vi "Get Bundler Input Terminal By Name.vi"(8 "error in (no error)":errorcluster, 10 "Terminal name":string, 11 "Bundler in":refnum<vi>) -> (0 "error out":errorcluster, 1 "Found?":bool, 2 "Terminal Refnum":refnum<vi>, 3 "Bundler out":refnum<vi>)   [LabVIEW 2019, in "gRPC Template Creation Utility.lvlib"]
uses:
  gRPC Template Creation Utility.lvlib
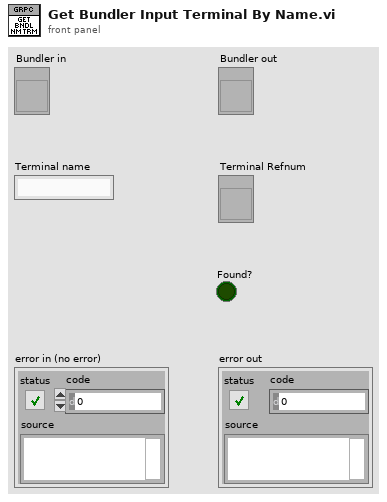
[diagram p1: front panel]
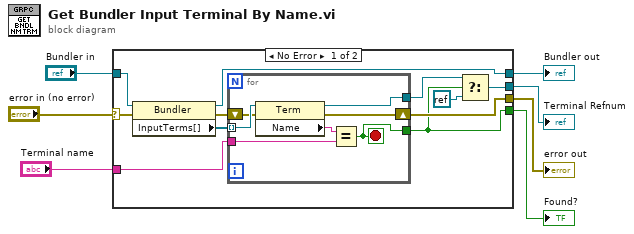
[diagram p0: block diagram]
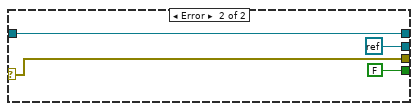
[diagram p2: hidden frame]
diagram:
  n1 = case shown="No Error" "error in (no error)" {
    selector: "error in (no error)" -> [w12 w26]
    tunnel: "Bundler in" -> [w16 w28]
    tunnel: [w15 w26] -> w6
    tunnel: "Terminal name" -> [w14 _]
    tunnel: [w11 FALSE] -> w4
    tunnel: [w8 refnum<k0> refnum] -> w3
    tunnel: [w13 w28] -> w2
    frame No Error {
      n2 = property class="Bundler"(reference=w16, error in=w12) -> (reference out=w13:refnum<vi>, error out=w18:errorcluster, "InputTerms[]"=w17:refnum<vi>[])
      n3 = for {
        tunnel: w17 -> [w25] mode=indexing
        shift-right: [w23] -> w15
        shift-left: w18 -> [w24]
        tunnel: w14 -> [w21]
        tunnel: [w20] -> w9
        tunnel: [w19] -> w11
        stop <- w19 stop-if-true
        n4 = property class="Term"(reference=w25, error in=w24) -> (reference out=w20:refnum<vi>, error out=w23:errorcluster, "Name"=w22:string)
        n5 = Equal?(x=w22, y=w21) -> (x = y?=w19:bool)
      }
      n6 = Select(t=w9, s=w11, f=refnum<k0> refnum) -> (s? t:f=w8:refnum<vi>)
    }
    frame Error {
    }
  }
  "error out" <- w6
  "Terminal Refnum" <- w3
  "Found?" <- w4
  "Bundler out" <- w2
